vi "oax_gsOrder Analyzer.vi"() -> ()   [LabVIEW 2017]
doc: "This VI provides Gabor order track, which can extract order from sound / vibration signal and playback on multimedia devices. This VI also provides access to Order Map.vi, which displays spectral maps, in menu bar window>> Show Order Map."
uses:
  <vilib>/addons/Sound and Vibration/Order Analysis/Ref Gabor Order Tracking/window information.ctl
  <vilib>/Analysis/1siggen.llb/Ramp Pattern by Samples.vi
  <vilib>/Waveform/WDTFileIO.llb/ Write Waveforms to File (1D).vi
  <vilib>/Waveform/WDTFileIO.llb/Export Waveforms To Spreadsheet File (1D).vi
  <vilib>/addons/Sound and Vibration/Order Analysis/Example Support/Demo VI/Start-Up Kit/OAT Start/global variable.vi
  <vilib>/addons/Sound and Vibration/Order Analysis/Ref Gabor Order Tracking/Get Freq-Time Spectral Map (U8).vi
  <vilib>/addons/Sound and Vibration/Order Analysis/Gabor Order Tracking/SoundVib_Gabor.lvlib
  <vilib>/Analysis/NI_AALBase.lvlib
panel:
  in  "Select Data":string(tree)="Runup.bin"
  in  "Campbell Diagram":bool
  in  "order map":bool
  in  "Save Orders":bool
  in  "Clear":bool
  in  "Delete":bool
  out "Speed at\nCursor (RPM)":dbl
  out "Time at\nCursor (sec)":dbl format="%.2f"
  in  "last path":path
  in  "unit":u16(ring) items=["Order", "Hz"]
  out "window information":T1={"window type"=3, "window length"=1} {"window type" items=["None"=0, "Hanning"=1, "Hamming"=2, "Blackman-Harris"=3, "Exact Blackman"=4, "Blackman"=5, "Flat Top"=6, "4 Term B-Harris"=7, "7 Term B-Harris"=8, "Low Sidelobe"=9, "Gaussian"=62]; "window length" min=0}
  out "TF Plot":u8[][](graph) caption="Time-Frequency Plot"
  out "Cursor Position":cluster{"Cursor X":dbl, "Cursor Y":dbl}={"Cursor X"=347.3140311804009, "Cursor Y"=0.0} {"Cursor Y" format="%.2f"; "Cursor X" format="%.2f"}
  in  "Play Sound":T2(ring)
  in  "Order List":i32[](listbox)
  out "Spectrum":cluster{dbl[], "X":dbl[]}(graph)
  out "mask":bool[][](array[boolean])
  in  "Bandwidth":dbl(slide)=0.5 min=0.0 scale=0.0..1.0 scale format="%.2f"
  in  "extract":bool
  out "X":dbl[](array[numeric]) format="%.2f"
  in  "Selected Order":dbl min=0.0 step=0.10000000149011612 format="%.1f"
  out "Window \nLength":i32
  out "Status":string="Waiting..."
  out "Sample \nRate (Hz)":dbl
  out "File Name":string
  out "S&V plot":dbl[][](graph)
  # "Show Other Formats"
  # "Extract Order Waveforms"
  # "Narrow"
  # "Wide"
  # "Status"
  # "Data Info"
  # "Cursor Values"
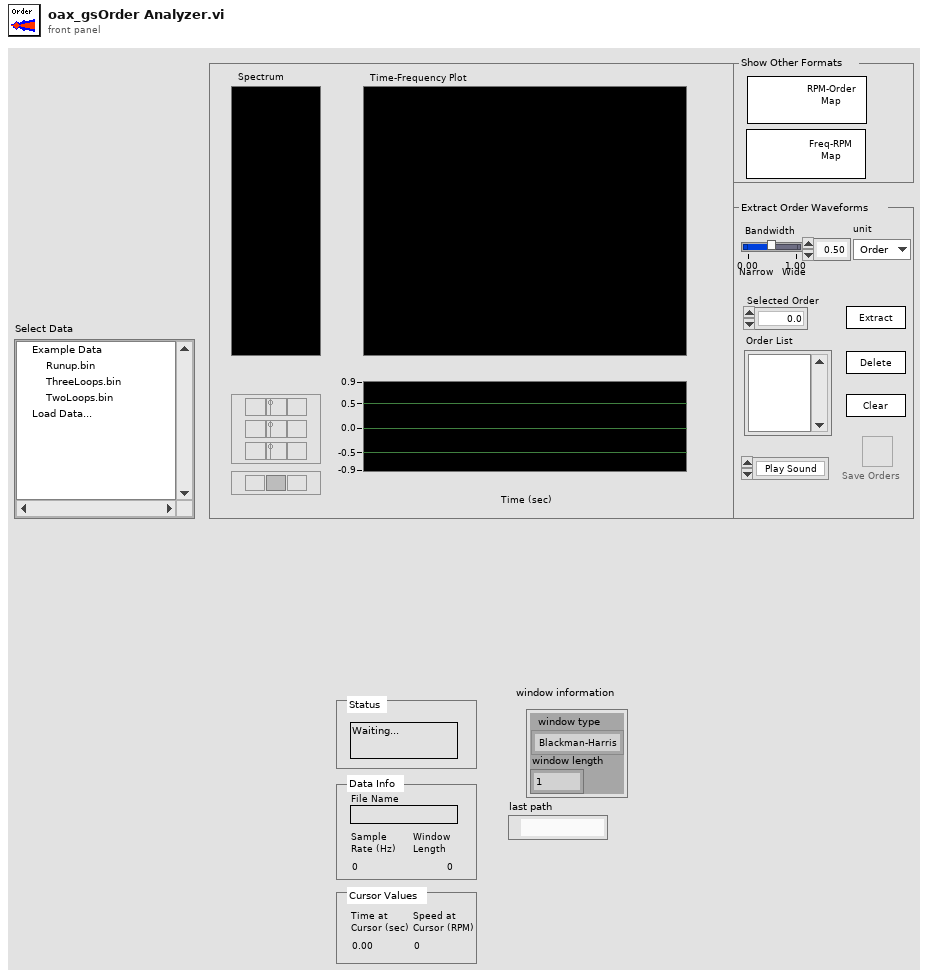
[diagram p1: front panel]
types:
  T1 = typedef "SoundVib_Gabor.lvlib/window information.ctl" = cluster{"window type":u32, "window length":i32}
  T2 = enum16{"Play Sound", "Original Signal", "Selected Orders", "Without Orders"}
  T3 = enum16{"Play Sound", "Original Samples", "Selected Orders", "Without Orders"}
  T4 = typedef "LVPointDoubleTypeDef.ctl" = cluster{"Cursor X":dbl, "Cursor Y":dbl}
  T5 = cluster{"Selected Order":dbl, "Bandwidth":dbl, "unit":u16}
  T6 = typedef "LVRangeTypeDef.ctl" = cluster{"Minimum":dbl, "Maximum":dbl, "Increment":dbl, "Minor Increment":dbl, "Start":dbl}
  T7 = typedef "SoundVib_Gabor.lvlib/GT RefNum.ctl" = refnum<k1>
  T8 = typedef "SoundVib_TachProcess.lvlib/speed profile.ctl" = cluster{"time [s]":dbl[], "speed [RPM]":dbl[]}
  T9 = cluster{"quality":enum16{"mono", "stereo"}, u32, "bits/sample":enum16{"8 bit", "16 bit"}}
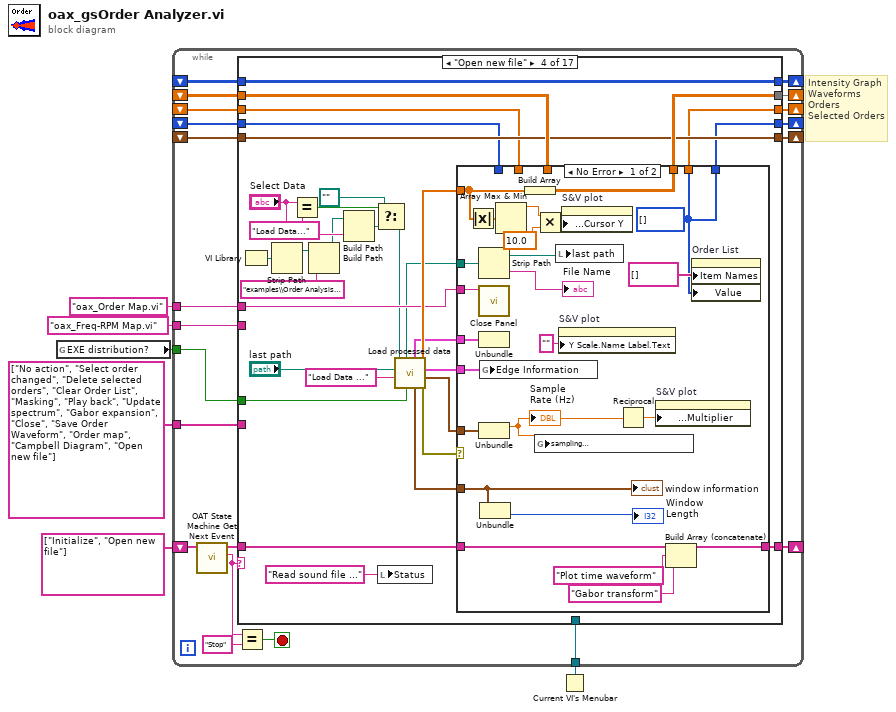
[diagram p0: block diagram]
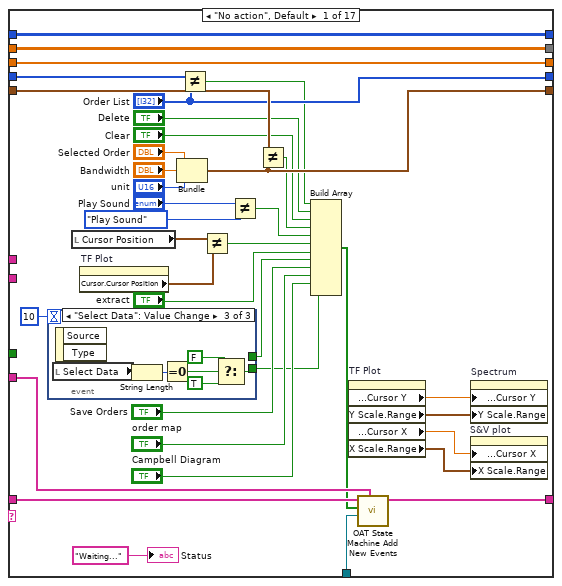
[diagram p2: hidden frame]
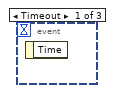
[diagram p3: hidden frame]
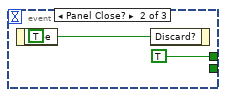
[diagram p4: hidden frame]
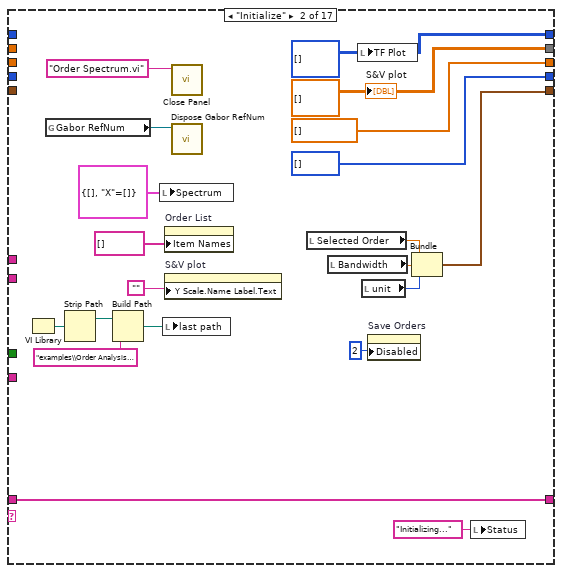
[diagram p5: hidden frame]
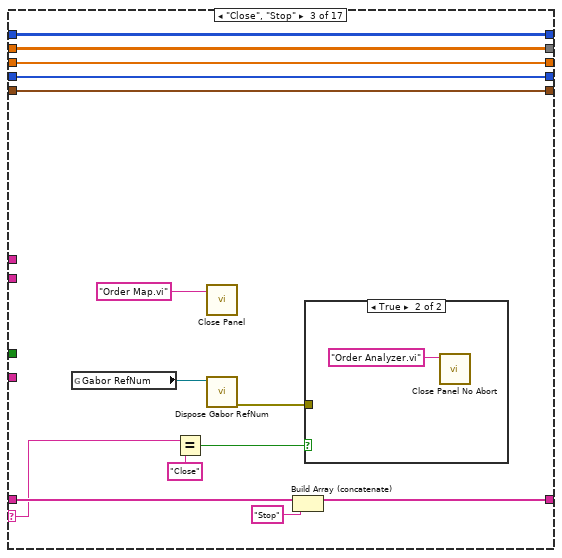
[diagram p6: hidden frame]
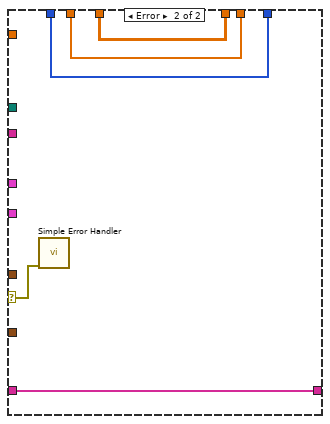
[diagram p8: hidden frame]
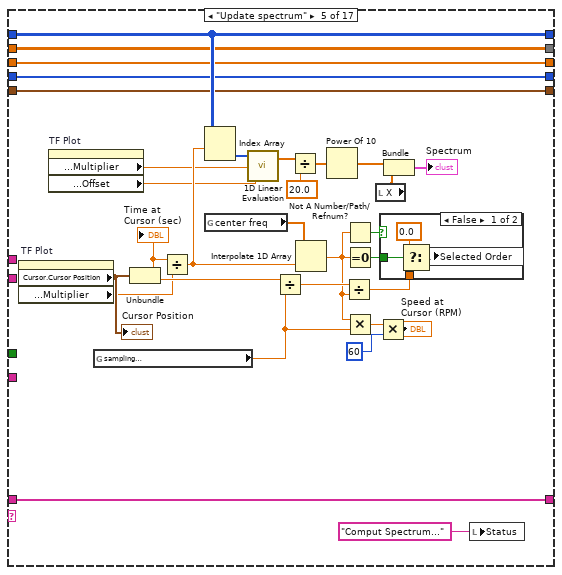
[diagram p9: hidden frame]
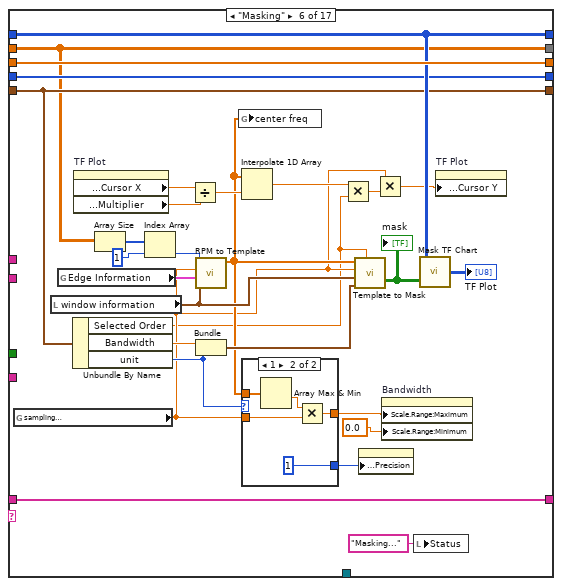
[diagram p11: hidden frame]
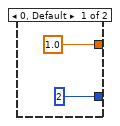
[diagram p12: hidden frame]
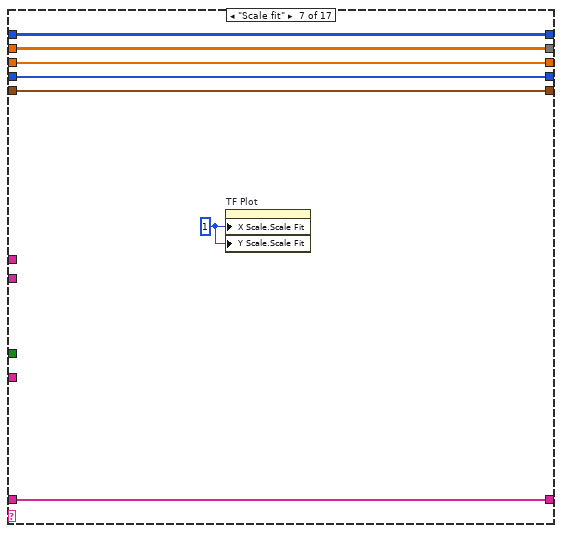
[diagram p13: hidden frame]
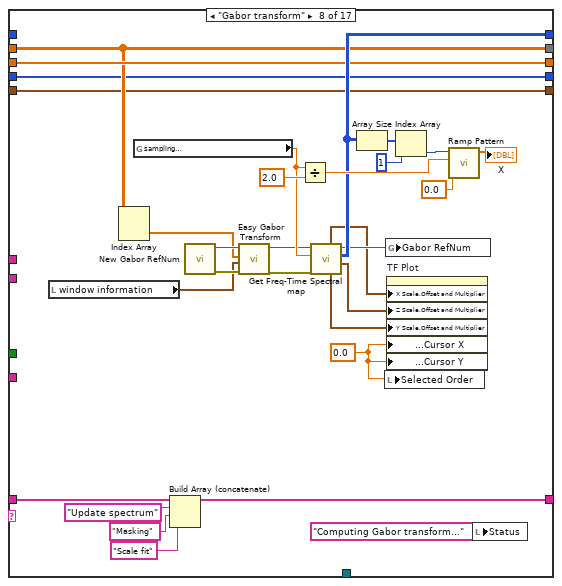
[diagram p14: hidden frame]
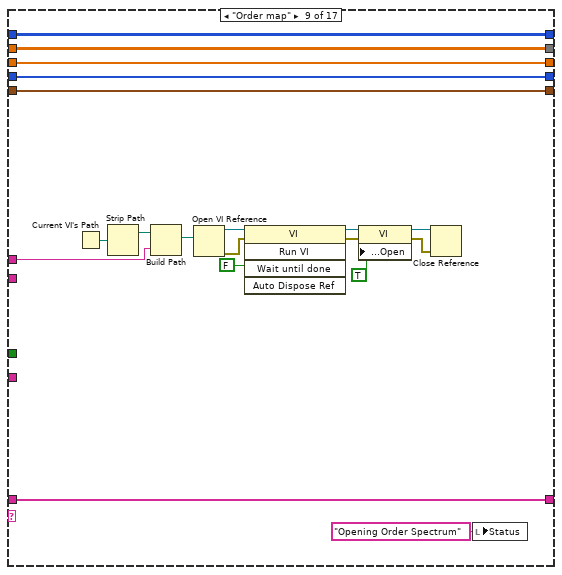
[diagram p15: hidden frame]
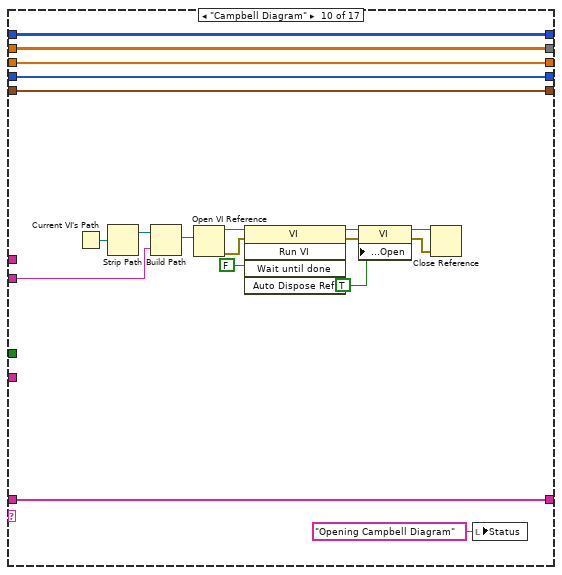
[diagram p16: hidden frame]
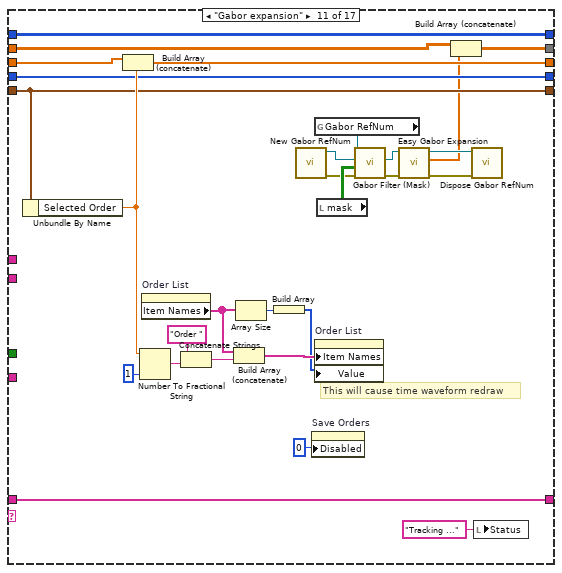
[diagram p17: hidden frame]
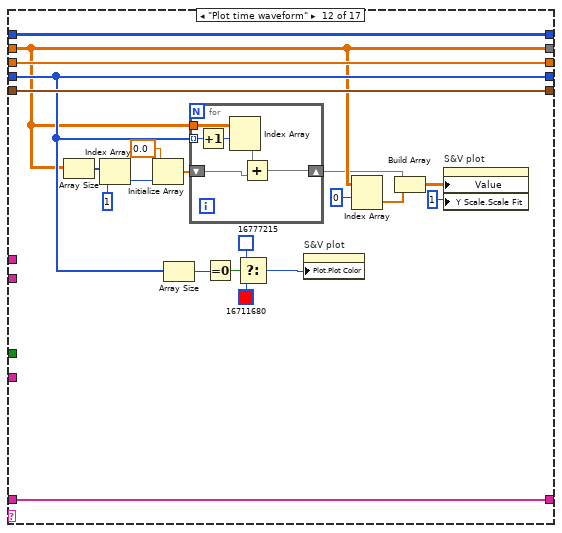
[diagram p18: hidden frame]
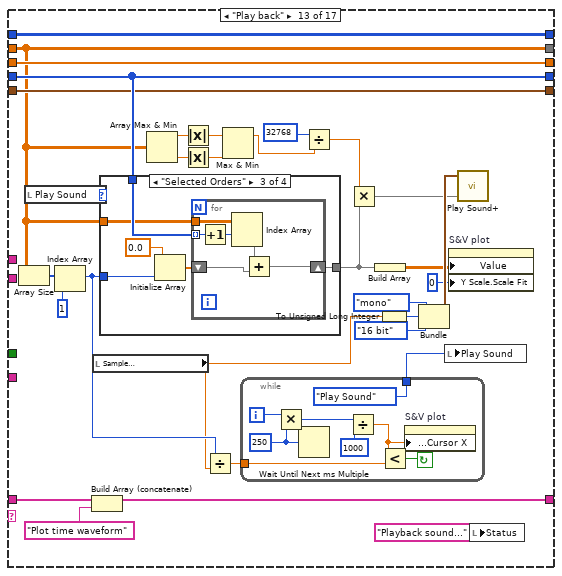
[diagram p19: hidden frame]
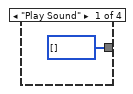
[diagram p20: hidden frame]
diagram:
  # "Intensity Graph\nWaveforms\nOrders\nSelected Orders"
  n1 = global read "global variable.vi" "EXE distribution?"() -> (w2:bool)
  n2 = Current VI's Menubar() -> (w4:refnum<k9>)
  n3 = while {
    tunnel: "oax_Freq-RPM Map.vi" ("VI name") -> [w7]
    tunnel: w2 -> [w8]
    tunnel: "oax_Order Map.vi" ("VI name") -> [w9]
    shift-left: _ -> [w11]
    shift-right: [w10] -> _
    shift-left: _ -> [w12]
    shift-right: [w13] -> _
    tunnel: w4 -> [w14]
    tunnel: string[] ["No action", "Select order changed", "Delete selected orders", "Clear Order List", "Masking", "Play back", "Update spectrum", "Gabor expansion", "Close", "Save Order Waveform", "Order map", "Campbell Diagram", "Open new file"] ("Event Queue Out") -> [w18]
    shift-left: string[] ["Initialize", "Open new file"] ("Event Queue Out") -> [w21]
    shift-right: [w19] -> _
    shift-left: _ -> [w22]
    shift-right: [w24] -> _
    shift-left: _ -> [w23]
    shift-right: [w25] -> _
    shift-left: _ -> [w26]
    shift-right: [w27] -> _
    stop <- w15 stop-if-true
    n4 = call <vilib>:"OAT State Machine Get Next Event.vi"("event queue in"=w21) -> ("next event"=w17:string, "event queue out"=w20:string[])  [unwired: 5 in]
    n5 = Equal?(x=w17, y="Stop" ("item tag")) -> (x = y?=w15:bool)
    n6 = case shown="\"Open new file\"" w17 {
      selector: w17 -> [_ _ w98 _ _ _ _ _ _ _ _ _ _ _ _ _ _]
      tunnel: [w64 w89 w106 w139 w199 w230 w243 w268 w295 w314 w339 w363 w400 w449 w466 w486 w498] -> w27
      tunnel: w26 -> [w64 _ w106 w139 w199 w230 w243 _ w295 w314 w339 w363 w400 w449 w466 w486 w498]
      tunnel: [w63 w80 w105 w135 w198 w223 w242 w265 w294 w313 w337 w347 w377 w443 w457 w485 w492] -> w25
      tunnel: [w62 dbl[] [] w104 w121 w197 w232 w246 w267 w293 w312 w329 w350 w399 w438 w455 w484 w497] -> w24
      tunnel: w23 -> [w63 _ w105 w134 w198 w223 w242 w265 w294 w313 w338 w347 w377 w444 w460 w485 w492]
      tunnel: w22 -> [w62 _ w104 w123 w197 w232 w246 w267 w293 w312 w335 w350 w399 _ w456 w484 w497]
      tunnel: w20 -> [w61 w86 w101 w131 w196 w211 w240 w262 w291 w310 w316 w357 w393 w448 w463 w480 w495]
      tunnel: [w60 w86 w94 w132 w196 w211 w240 w261 w291 w310 w316 w357 w391 w445 w462 w479 w495] -> w19
      tunnel: w18 -> [w59 _ _ _ _ _ _ _ _ _ _ _ _ _ _ _ _]
      tunnel: w14 -> [w57 _ _ _ _ _ _ _ _ _ _ _ _ _ _ _ _]
      tunnel: [w56 w81 w102 w130 w193 w226 w245 w256 w288 w307 w321 w356 w381 w442 w465 w482 w496] -> w13
      tunnel: w12 -> [w55 _ w102 w130 w193 w226 w245 w256 w288 w307 w321 w356 w381 w442 w465 w482 w496]
      tunnel: w11 -> [w36 _ w103 w122 w194 w225 w244 w257 w289 w308 w322 w348 w389 w441 w459 w483 w491]
      tunnel: ["Order List" i32[] [] ("Order List") w103 w120 w194 w225 w244 w257 w289 w308 w322 w348 w389 w441 i32[] [] ("Order List") w483 w491] -> w10
      tunnel: w9 -> [_ _ _ w125 _ _ _ _ w277 _ _ _ _ _ _ _ _]
      tunnel: w8 -> [_ _ _ w119 _ _ _ _ _ _ _ _ _ _ _ _ _]
      tunnel: w7 -> [_ _ _ _ _ _ _ _ _ w296 _ _ _ _ _ _ _]
      frame "No action", Default {
        n7 = event shown="[2] \"Select Data\": Value Change" {
          selector: _ -> [_ _ _]
          dyn-events: _ -> [_ _ _]
          timeout: 10 -> [_ _ _]
          tunnel: [_ TRUE _] -> w32
          tunnel: [_ _ w68] -> w28
          event Timeout {
            n8 = event-data() -> ()  [unwired: 1 in, 1 out]
          }
          event Panel Close? {
            n9 = event-data() -> ()  [unwired: 1 in, 1 out]
            n10 = event-data("Discard?"=TRUE) -> ()  [unwired: 1 in, 1 out]
          }
          event "Select Data": Value Change {
            n11 = local read "Select Data"() -> (w72:string)
            n12 = event-data() -> ()  [unwired: 1 in, 2 out]
            n13 = String Length(string=w72) -> (length=w71:i32)
            n14 = Equal To 0?(x=w71) -> (x = 0?=w70:bool)
            n15 = Select(t=FALSE, s=w70, f=TRUE) -> (s? t:f=w68:bool)
          }
        }
        n16 = local read "Cursor Position"() -> (w53:cluster{"Cursor X":dbl, "Cursor Y":dbl})
        n17 = property on="TF Plot" class="IntGraph (strict)"() -> ("Cursor.Cursor Position"=w52:T4)  [unwired: 2 in, 2 out]
        n18 = Bundle("Selected Order"="Selected Order", "Bandwidth"="Bandwidth", "unit"="unit") -> (w56:T5)  [unwired: 1 in]
        n19 = Not Equal?(x=w36, y="Order List") -> (x != y?=w34:bool)
        n20 = Not Equal?(x=w53, y=w52) -> (x != y?=w45:bool)
        n21 = Not Equal?(x="Play Sound", y=T3."Play Sound" ("play sound")) -> (x != y?=w42:bool)
        n22 = Not Equal?(x=w55, y=w56) -> (x != y?=w46:bool)
        n23 = Build Array(w34, "Delete", "Clear", w46, w42, w45, "extract", w32, "Save Orders", "order map", "Campbell Diagram", w28) -> (w54:bool[])
        n24 = property on="TF Plot" class="IntGraph (strict)"() -> ("Cursor.Cursor Position:Cursor Y"=w49:dbl, "Y Scale.Range"=w50:T6, "Cursor.Cursor Position:Cursor X"=w39:dbl, "X Scale.Range"=w40:T6)  [unwired: 2 in, 2 out]
        n25 = call <vilib>:"OAT State Machine Add New Events.vi"("Event Names"=w59, "Menu Refnum"=w57, "New Events"=w54, "Event Queue In"=w61) -> ("Event Queue Out"=w60:string[])  [unwired: 7 in]
        n26 = property on="Spectrum" class="XYGraph (strict)"("Cursor.Cursor Position:Cursor Y"=w49, "Y Scale.Range"=w50) -> ()  [unwired: 2 in, 2 out]
        n27 = property on="S&V plot" class="WFGraph (strict)"("Cursor.Cursor Position:Cursor X"=w39, "X Scale.Range"=w40) -> ()  [unwired: 2 in, 2 out]
        "Status" <- "Waiting..." ("status")
      }
      frame "Initialize" {
        w80 = dbl[][] []
        w89 = u8[][] [] ("graph [U8]")
        n28 = VI Library() -> (path=w78:path)
        n29 = global read "global variable.vi" "Gabor RefNum"() -> (w90:T7)
        n30 = Strip Path(path=w78) -> (stripped path=w77:path)  [unwired: 1 out]
        n31 = Build Path(base path=w77, name or relative path="examples\\Order Analysis\\Demo VI\\Example Data") -> (appended path=w75:path)
        n32 = local write "Spectrum"(cluster{dbl[], "X":dbl[]} {[], "X"=[]} ("Instantaneous\nSpectrum")) -> ()
        n33 = local write "last path"(w75) -> ()
        n34 = property on="Order List" class="LstBox (strict)"("Item Names"=string[] [] ("Write Attribute")) -> ()  [unwired: 2 in, 2 out]
        n35 = property on="S&V plot" class="WFGraph (strict)"("Y Scale.Name Label.Text"="") -> ()  [unwired: 2 in, 2 out]
        n36 = call <vilib>:"Close Panel.vi"("VI name"="Order Spectrum.vi") -> ()  [unwired: 10 in, 1 out]
        n37 = call <vilib>:"Dispose Gabor RefNum.vi"("RefNum in"=w90) -> ()  [unwired: 7 in, 1 out]
        n38 = local read "Selected Order"() -> (w83:dbl)
        n39 = local read "Bandwidth"() -> (w82:dbl)
        n40 = local write "TF Plot"(w89) -> ()
        n41 = local read "unit"() -> (w79:u16)
        n42 = property on="Save Orders" class="Bool"("Disabled"=u8 2) -> ()  [unwired: 2 in, 2 out]
        n43 = Bundle("Selected Order"=w83, "Bandwidth"=w82, "unit"=w79) -> (w81:T5)  [unwired: 1 in]
        n44 = local write "Status"("Initializing..." ("status")) -> ()
        "S&V plot" <- w80
      }
      frame "Close", "Stop" {
        n45 = global read "global variable.vi" "Gabor RefNum"() -> (w100:T7)
        n46 = Equal?(x=w98, y="Close") -> (x = y?=w96:bool)
        n47 = call <vilib>:"Close Panel.vi"("VI name"="Order Map.vi") -> ()  [unwired: 10 in, 1 out]
        n48 = call <vilib>:"Dispose Gabor RefNum.vi"("RefNum in"=w100) -> ("error out"=w95:errorcluster)  [unwired: 7 in]
        n49 = Build Array (concatenate)(w101, "Stop") -> (w94:string[])
        n50 = case shown="True" w96 {
          tunnel: w95 -> [_ _]
          frame False {
          }
          frame True {
            n51 = call <vilib>:"Close Panel No Abort.vi"("VI name"="Order Analyzer.vi") -> ()  [unwired: 10 in, 1 out]
          }
        }
      }
      frame "Open new file" {
        n52 = VI Library() -> (path=w111:path)
        n53 = Strip Path(path=w111) -> (stripped path=w110:path)  [unwired: 1 out]
        n54 = Equal?(x="Select Data", y="Load Data...") -> (x = y?=w114:bool)
        n55 = Build Path(base path=w110, name or relative path="examples\\Order Analysis\\Demo VI\\Example Data") -> (appended path=w108:path)
        n56 = Build Path(base path=w108, name or relative path="Select Data") -> (appended path=w113:path)
        n57 = Select(t=path "" ("last path"), s=w114, f=w113) -> (s? t:f=w112:path)
        n58 = local write "Status"("Read sound file ..." ("status")) -> ()
        n59 = call <vilib>:"Load processed data.vi"("EXE distribution?"=w119, "Prompt"="Load Data ...", "start path"="last path", "file path"=w112) -> ("error out"=w136:errorcluster, "parameters"=w127:cluster{"sample rate":sgl, "pulses/rev":i32}, "speed profile"=w138:T8, "S&V samples"=w129:dbl[], "window info"=w126:T1, "lables"=w128:cluster{"tach lable":string, "S&V lable":string}, "file path out"=w124:path)  [unwired: 1 in]
        n60 = case shown="No Error" w136 {
          selector: w136 -> [_ w166]
          tunnel: w124 -> [w161 _]
          tunnel: w138 -> [w160 _]
          tunnel: w127 -> [w155 _]
          tunnel: w129 -> [w145 _]
          tunnel: [w158 w168] -> w135
          tunnel: w134 -> [_ w168]
          tunnel: [w157 w167] -> w132
          tunnel: w131 -> [w156 w167]
          tunnel: w128 -> [w153 _]
          tunnel: w126 -> [w150 _]
          tunnel: w125 -> [w163 _]
          tunnel: w123 -> [_ w165]
          tunnel: w122 -> [_ w164]
          tunnel: [w146 w165] -> w121
          tunnel: [w146 w164] -> w120
          frame No Error {
            w146 = i32[] [] ("Order List")
            n61 = Absolute Value(x=w145) -> (abs(x)=w144:dbl[])
            n62 = Strip Path(path=w161) -> (stripped path=w148:path, name=→"File Name":string)
            n63 = call <vilib>:"Close Panel.vi"("VI name"=w163) -> ()  [unwired: 10 in, 1 out]
            n64 = Unbundle(w153) -> ()  [unwired: 2 out]
            n65 = Unbundle(w155) -> ("sample rate"=w154:sgl)  [unwired: 1 out]
            "Sample \nRate (Hz)" <- w154
            n66 = global write "global variable.vi" "Edge Information"(w160) -> ()
            n67 = Unbundle(w150) -> ("window length"=→"Window \nLength":i32)  [unwired: 1 out]
            n68 = Array Max & Min(array=w144) -> (max value=w143:dbl)  [unwired: 3 out]
            n69 = Build Array(w145) -> (w158:dbl[][])
            n70 = Multiply(x=w143, y=10.0) -> (x*y=w141:dbl)
            n71 = global write "global variable.vi" "sampling \nfrequency (Hz)"(w154) -> ()
            n72 = local write "last path"(w148) -> ()
            n73 = property on="S&V plot" class="WFGraph (strict)"("Y Scale.Name Label.Text"="") -> ()  [unwired: 2 in, 2 out]
            n74 = property on="S&V plot" class="WFGraph (strict)"("Cursor.Cursor Position:Cursor Y"=w141) -> ()  [unwired: 2 in, 2 out]
            n75 = Reciprocal(x=w154) -> (1/x=w159:sgl)
            n76 = property on="S&V plot" class="WFGraph (strict)"("X Scale.Offset and Multiplier:Multiplier"=w159) -> ()  [unwired: 2 in, 2 out]
            n77 = Build Array (concatenate)(w156, "Plot time waveform" ("status"), "Gabor transform" ("status")) -> (w157:string[])
            n78 = property on="Order List" class="LstBox (strict)"("Item Names"=string[] [], "Value"=w146) -> ()  [unwired: 2 in, 2 out]
            "window information" <- w150
          }
          frame Error {
            n79 = call <vilib>:"Simple Error Handler.vi"("error in (no error)"=w166) -> ()  [unwired: 4 in, 5 out]
          }
        }
      }
      frame "Update spectrum" {
        n80 = property on="TF Plot" class="IntGraph (strict)"() -> ("Cursor.Cursor Position"=w187:T4, "X Scale.Offset and Multiplier:Multiplier"=w184:dbl)  [unwired: 2 in, 2 out]
        "Cursor Position" <- w187
        n81 = property on="TF Plot" class="IntGraph (strict)"() -> ("Z Scale.Offset and Multiplier:Multiplier"=w179:dbl, "Z Scale.Offset and Multiplier:Offset"=w178:dbl)  [unwired: 2 in, 2 out]
        n82 = global read "global variable.vi" "sampling \nfrequency (Hz)"() -> (w171:dbl)
        n83 = Unbundle(w187) -> ("Cursor X"=w173:dbl, "Cursor Y"=w186:dbl)
        "Time at\nCursor (sec)" <- w173
        n84 = Divide(x=w173, y=w184) -> (x/y=w185:dbl)
        n85 = Index Array(array=w199, index (row)=w185) -> (element=w183:u8[])  [unwired: 1 in]
        n86 = global read "global variable.vi" "center freq"() -> (w177:dbl[])
        n87 = call <vilib>:"1D Linear Evaluation.vi"("offset"=w178, "scale"=w179, "X"=w183) -> ("Y[i]=X[i]*a+b"=w182:dbl[])  [unwired: 1 out]
        n88 = Divide(x=w186, y=w171) -> (x/y=w189:dbl)
        n89 = Divide(x=w182, y=20.0 ("Write Attribute")) -> (x/y=w181:dbl[])
        n90 = Interpolate 1D Array(1:w185, 2:w177) -> (0:w176:dbl)
        n91 = Power Of 10(x=w181) -> (10^x=w190:dbl[])
        n92 = Divide(x=w189, y=w176) -> (x/y=w188:dbl)
        n93 = Not A Number/Path/Refnum?(number/path/refnum=w176) -> (NaN/Path/Refnum?=w169:bool)
        n94 = Equal To 0?(x=w176) -> (x = 0?=w170:bool)
        n95 = Multiply(x=w176, y=w171) -> (x*y=w172:dbl)
        n96 = local read "X"() -> (w191:dbl[])
        n97 = Multiply(x=w172, y=60) -> (x*y=→"Speed at\nCursor (RPM)":dbl)
        n98 = case shown="False" w169 {
          tunnel: w188 -> [w203 _]
          tunnel: w170 -> [w200 _]
          frame False {
            n99 = Select(t=0.0, s=w200, f=w203) -> (s? t:f=w201:dbl)
            n100 = local write "Selected Order"(w201) -> ()
          }
          frame True {
          }
        }
        n101 = Bundle(w190, "X"=w191) -> (→"Spectrum":cluster{dbl[], "X":dbl[]})  [unwired: 1 in]
        n102 = local write "Status"("Comput Spectrum..." ("status")) -> ()
      }
      frame "Masking" {
        n103 = global read "global variable.vi" "sampling \nfrequency (Hz)"() -> (w209:dbl)
        n104 = local read "window information"() -> (w218:T1)
        n105 = global read "global variable.vi" "Edge Information"() -> (w224:T8)
        n106 = Unbundle By Name(w226) -> ("Selected Order"=w208:dbl, "Bandwidth"=w217:dbl, "unit"=w216:u16)
        n107 = property on="TF Plot" class="IntGraph (strict)"() -> ("Cursor.Cursor Position:Cursor X"=w231:dbl, "X Scale.Offset and Multiplier:Multiplier"=w227:dbl)  [unwired: 2 in, 2 out]
        n108 = Array Size(array=w223) -> (size(s)=w222:i32[])
        n109 = Index Array(array=w222, index=1 ("Index")) -> (element=w221:i32)
        n110 = Divide(x=w231, y=w227) -> (x/y=w228:dbl)
        n111 = call <vilib>:"RPM to Template.vi"("window info"=w218, "speed profile"=w224, "sampling frequency [Hz]"=w209, "signal length"=w221) -> ("Gabor template"=w214:dbl[])  [unwired: 6 in, 1 out]
        n112 = Bundle("Bandwidth"=w217, "unit"=w216) -> (w215:cluster{"Bandwidth":dbl, "unit":u16})  [unwired: 1 in]
        n113 = global write "global variable.vi" "center freq"(w214) -> ()
        n114 = Interpolate 1D Array(1:w228, 2:w214) -> (0:w220:dbl)
        n115 = case shown="1" w216 {
          tunnel: w214 -> [_ w239]
          tunnel: w209 -> [_ w237]
          tunnel: [1.0 w236] -> w213
          tunnel: [u8 2 u8 1] -> w212
          frame 0, Default {
          }
          frame 1 {
            n116 = Array Max & Min(array=w239) -> (min value=w238:dbl)  [unwired: 3 out]
            n117 = Multiply(x=w238, y=w237) -> (x*y=w236:dbl)
          }
        }
        n118 = Multiply(x=w220, y=w208) -> (x*y=w204:dbl)
        n119 = call <vilib>:"Template to Mask.vi"("order (1.0)"=w208, "bandwidth"=w215, "window info"=w218, "sampling frequency [S/s]"=w209, "Gabor template"=w214) -> ("mask array"=w206:bool[][])  [unwired: 6 in]
        "mask" <- w206
        n120 = property class="DigNum (strict)"("Format & Precision:Precision"=w212) -> ()  [unwired: 2 in, 2 out]
        n121 = Multiply(x=w209, y=w204) -> (x*y=w207:dbl)
        n122 = property on="Bandwidth" class="Slide (strict)"("Scale.Range:Maximum"=w213, "Scale.Range:Minimum"=0.0) -> ()  [unwired: 2 in, 2 out]
        n123 = local write "Status"("Masking..." ("status")) -> ()
        n124 = call <vilib>:"Mask TF Chart.vi"("Mask Array"=w206, "TF plot"=w230) -> ("TF plot Out"=→"TF Plot":u8[][])
        n125 = property on="TF Plot" class="IntGraph (strict)"("Cursor.Cursor Position:Cursor Y"=w207) -> ()  [unwired: 2 in, 2 out]
      }
      frame "Scale fit" {
        w241 = u8 1 ("X Scale.Scale Fit")
        n126 = property on="TF Plot" class="IntGraph (strict)"("X Scale.Scale Fit"=w241, "Y Scale.Scale Fit"=w241) -> ()  [unwired: 2 in, 2 out]
      }
      frame "Gabor transform" {
        w247 = 0.0
        n127 = local read "window information"() -> (w255:T1)
        n128 = Index Array(array=w265) -> (element=w263:dbl[])  [unwired: 2 in]
        n129 = global read "global variable.vi" "sampling \nfrequency (Hz)"() -> (w254:dbl)
        n130 = Build Array (concatenate)(w262, "Update spectrum" ("status"), "Masking" ("status"), "Scale fit" ("status")) -> (w261:string[])
        n131 = call <vilib>:"New Gabor RefNum.vi"() -> ("error out"=w264:errorcluster, "RefNum"=w276:T7)  [unwired: 9 in]
        n132 = call <vilib>:"Easy Gabor Transform.vi"("error in (no error)"=w264, "window info"=w255, "x[n]"=w263, "RefNum in"=w276) -> ("error out"=w275:errorcluster, "RefNum out"=w253:T7)  [unwired: 3 in, 3 out]
        n133 = Divide(x=w254, y=2.0) -> (x/y=w270:dbl)
        n134 = call-poly <vilib>:"Get Freq-Time Spectral map.vi"("error in (no error)"=w275, "sampling frequency [Hz]"=w254, "RefNum in"=w253) -> ("quantization info"=w250:cluster{"offset":dbl, "multiplier":dbl}, "spectral map"=w268:u8[][], "RefNum out"=w266:T7, "frequency scale"=w249:cluster{"offset":dbl, "multiplier":dbl}, "time scale"=w251:cluster{"offset":dbl, "multiplier":dbl})  [unwired: 3 in, 1 out]
        n135 = Array Size(array=w268) -> (size(s)=w274:i32[])
        n136 = local write "Selected Order"(w247) -> ()
        n137 = global write "global variable.vi" "Gabor RefNum"(w266) -> ()
        n138 = property on="TF Plot" class="IntGraph (strict)"("X Scale.Offset and Multiplier"=w251, "Z Scale.Offset and Multiplier"=w250, "Y Scale.Offset and Multiplier"=w249, "Cursor.Cursor Position:Cursor X"=w247, "Cursor.Cursor Position:Cursor Y"=w247) -> ()  [unwired: 2 in, 2 out]
        n139 = Index Array(array=w274, index=1 ("Index")) -> (element=w272:i32)
        n140 = call-poly <vilib>:"Ramp Pattern.vi"("start"=0.0, "end"=w270, "samples"=w272) -> ("Ramp Pattern"=→"X":dbl[])  [unwired: 7 in, 1 out]
        n141 = local write "Status"("Computing Gabor transform..." ("status")) -> ()
      }
      frame "Order map" {
        n142 = Current VI's Path() -> (path=w292:path)
        n143 = Strip Path(path=w292) -> (stripped path=w287:path)  [unwired: 1 out]
        n144 = Build Path(base path=w287, name or relative path=w277) -> (appended path=w286:path)
        n145 = Open VI Reference(vi path=w286) -> (vi reference=w285:refnum<vi>, error out=w284:errorcluster)  [unwired: 5 in]
        n146 = invoke class="VI" method="Run VI"(reference=w285, error in=w284, "Wait until done"=FALSE) -> (reference out=w282:refnum<vi>, error out=w281:errorcluster)  [unwired: 2 in, 3 out]
        n147 = property class="VI"(reference=w282, error in=w281, "Front Panel Window:Open"=TRUE) -> (reference out=w278:refnum<vi>, error out=w279:errorcluster)
        n148 = Close Reference(reference=w278, error in (no error)=w279) -> ()  [unwired: 1 out]
        n149 = local write "Status"("Opening Order Spectrum" ("status")) -> ()
      }
      frame "Campbell Diagram" {
        n150 = Current VI's Path() -> (path=w311:path)
        n151 = Strip Path(path=w311) -> (stripped path=w306:path)  [unwired: 1 out]
        n152 = Build Path(base path=w306, name or relative path=w296) -> (appended path=w305:path)
        n153 = Open VI Reference(vi path=w305) -> (vi reference=w304:refnum<vi>, error out=w303:errorcluster)  [unwired: 5 in]
        n154 = invoke class="VI" method="Run VI"(reference=w304, error in=w303, "Wait until done"=FALSE) -> (reference out=w301:refnum<vi>, error out=w300:errorcluster)  [unwired: 2 in, 3 out]
        n155 = property class="VI"(reference=w301, error in=w300, "Front Panel Window:Open"=TRUE) -> (reference out=w297:refnum<vi>, error out=w298:errorcluster)
        n156 = Close Reference(reference=w297, error in (no error)=w298) -> ()  [unwired: 1 out]
        n157 = local write "Status"("Opening Campbell Diagram" ("status")) -> ()
      }
      frame "Gabor expansion" {
        # "This will cause time waveform redraw"
        n158 = Unbundle By Name(w321) -> ("Selected Order"=w323:dbl)
        n159 = Build Array (concatenate)(w335, w323) -> (w329:dbl[])
        n160 = Number To Fractional String(number=w323, precision (6)=i16 1) -> (F-format string=w333:string)  [unwired: 2 in]
        n161 = property on="Order List" class="LstBox (strict)"() -> ("Item Names"=w319:string[])  [unwired: 2 in, 2 out]
        n162 = Concatenate Strings("Order " ("Substring"), w333) -> (w330:string)
        n163 = Build Array (concatenate)(w319, w330) -> (w328:string[])
        n164 = Array Size(array=w319) -> (size(s)=w317:i32)
        n165 = Build Array(w317) -> (w318:i32[])
        n166 = call <vilib>:"New Gabor RefNum.vi"() -> ("error out"=w325:errorcluster, "RefNum"=w341:T7)  [unwired: 9 in]
        n167 = property on="Save Orders" class="Bool"("Disabled"=u8 0) -> ()  [unwired: 2 in, 2 out]
        n168 = global read "global variable.vi" "Gabor RefNum"() -> (w331:T7)
        n169 = property on="Order List" class="LstBox (strict)"("Item Names"=w328, "Value"=w318) -> ()  [unwired: 2 in, 2 out]
        n170 = local read "mask"() -> (w336:bool[][])
        n171 = call <vilib>:"Gabor Filter (Mask).vi"("error in (no error)"=w325, "mask array"=w336, "dest RefNum in"=w341, "src RefNum in"=w331) -> ("error out"=w326:errorcluster, "dest RefNum out"=w342:T7)  [unwired: 5 in, 1 out]
        n172 = call <vilib>:"Easy Gabor Expansion.vi"("error in (no error)"=w326, "RefNum in"=w342) -> ("error out"=w327:errorcluster, "time waveform"=w320:dbl[], "RefNum out"=w340:T7)  [unwired: 7 in]
        n173 = Build Array (concatenate)(w338, w320) -> (w337:dbl[][])
        n174 = call <vilib>:"Dispose Gabor RefNum.vi"("error in (no error)"=w327, "RefNum in"=w340) -> ()  [unwired: 6 in, 1 out]
        n175 = local write "Status"("Tracking ..." ("status")) -> ()
      }
      frame "Plot time waveform" {
        n176 = Array Size(array=w347) -> (size(s)=w353:i32[])
        n177 = Index Array(array=w353, index=1 ("Index")) -> (element=w349:i32)
        n178 = Initialize Array(0.0 ("y"), w349) -> (w346:dbl[])
        n179 = Array Size(array=w348) -> (size(s)=w358:i32)
        n180 = for {
          tunnel: w347 -> [w368]
          tunnel: w348 -> [w367] mode=indexing
          shift-right: [w366] -> w344
          shift-left: w346 -> [w365]
          n181 = Increment(x=w367) -> (x+1=w369:i32)
          n182 = Index Array(array=w368, index (row)=w369) -> (element=w364:dbl[])  [unwired: 1 in]
          n183 = Add(x=w364, y=w365) -> (x+y=w366:dbl[])
        }
        n184 = Equal To 0?(x=w358) -> (x = 0?=w359:bool)
        n185 = Select(t=u32 16777215 ("Read Attribute"), s=w359, f=u32 16711680 ("Read Attribute")) -> (s? t:f=w362:u32)
        n186 = property on="S&V plot" class="WFGraph (strict)"("Plot.Plot Color"=w362) -> ()  [unwired: 2 in, 2 out]
        n187 = Index Array(array=w347, index (row)=0) -> (element=w343:dbl[])  [unwired: 1 in]
        n188 = Build Array(w344, w343) -> (w355:dbl[][])
        n189 = property on="S&V plot" class="WFGraph (strict)"("Value"=w355, "Y Scale.Scale Fit"=u8 1) -> ()  [unwired: 2 in, 2 out]
      }
      frame "Play back" {
        n190 = Array Size(array=w377) -> (size(s)=w376:i32[])
        n191 = local read "Play Sound"() -> (w388:T2)
        n192 = Index Array(array=w376, index=1 ("Index")) -> (element=w375:i32)
        n193 = Build Array (concatenate)(w393, "Plot time waveform" ("status")) -> (w391:string[])
        n194 = local read "Sample \nRate (Hz)"() -> (w374:dbl)
        n195 = case shown="\"Selected Orders\"" w388 {
          tunnel: w389 -> [_ _ w418 w429]
          tunnel: [i16[] [] w410 w417 w428] -> w380
          tunnel: w377 -> [_ w412 w416 w427]
          tunnel: w375 -> [_ _ w413 _]
          frame "Play Sound" {
          }
          frame "Original Signal" {
            n196 = Index Array(array=w412, index (row)=0 ("Index")) -> (element=w410:dbl[])  [unwired: 1 in]
          }
          frame "Selected Orders" {
            n197 = Initialize Array(0.0 ("y"), w413) -> (w415:dbl[])
            n198 = for {
              tunnel: w416 -> [w423]
              tunnel: w418 -> [w422] mode=indexing
              shift-right: [w421] -> w417
              shift-left: w415 -> [w420]
              n199 = Increment(x=w422) -> (x+1=w424:i32)
              n200 = Index Array(array=w423, index (row)=w424) -> (element=w419:dbl[])  [unwired: 1 in]
              n201 = Add(x=w419, y=w420) -> (x+y=w421:dbl[])
            }
          }
          frame "Without Orders" {
            n202 = Index Array(array=w427, index (row)=0 ("Index")) -> (element=w425:dbl[])  [unwired: 1 in]
            n203 = for {
              tunnel: w427 -> [w434]
              tunnel: w429 -> [w433] mode=indexing
              shift-right: [w431] -> w428
              shift-left: w425 -> [w432]
              n204 = Increment(x=w433) -> (x+1=w435:i32)
              n205 = Index Array(array=w434, index (row)=w435) -> (element=w430:dbl[])  [unwired: 1 in]
              n206 = Subtract(x=w432, y=w430) -> (x-y=w431:dbl[])
            }
          }
        }
        n207 = Array Max & Min(array=w377) -> (max value=w387:dbl, min value=w386:dbl)  [unwired: 2 out]
        n208 = Absolute Value(x=w387) -> (abs(x)=w385:dbl)
        n209 = Absolute Value(x=w386) -> (abs(x)=w384:dbl)
        n210 = Divide(x=w375, y=w374) -> (x/y=w398:dbl)
        n211 = Max & Min(x=w385, y=w384) -> (max(x,y)=w382:dbl)  [unwired: 1 out]
        n212 = while {
          tunnel: [T2."Play Sound" ("play sound")] -> w373
          tunnel: w398 -> [w403]
          i -> [w407]
          stop <- w402 continue-if-true
          w406 = u32 250 ("milliseconds to wait")
          n213 = Multiply(x=w407, y=w406) -> (x*y=w408:u32)
          n214 = Wait Until Next ms Multiple(millisecond multiple=w406) -> ()  [unwired: 1 out]
          n215 = Divide(x=w408, y=u32 1000) -> (x/y=w404:dbl)
          n216 = Less?(x=w404, y=w403) -> (x < y?=w402:bool)
          n217 = property on="S&V plot" class="WFGraph (strict)"("Cursor.Cursor Position:Cursor X"=w404) -> ()  [unwired: 2 in, 2 out]
        }
        n218 = Divide(x=32768, y=w382) -> (x/y=w379:dbl)
        n219 = Multiply(x=w379, y=w380) -> (x*y=w378:dbl[])
        n220 = Build Array(w380) -> (w372:dbl[][])
        n221 = To Unsigned Long Integer(number=w374) -> (unsigned 32bit integer=w394:u32)
        n222 = Bundle("quality"=enum16{"mono", "stereo"}."mono", w394, "bits/sample"=enum16{"8 bit", "16 bit"}."16 bit") -> (w397:T9)  [unwired: 1 in]
        n223 = local write "Play Sound"(w373) -> ()
        n224 = property on="S&V plot" class="WFGraph (strict)"("Value"=w372, "Y Scale.Scale Fit"=u8 0) -> ()  [unwired: 2 in, 2 out]
        n225 = call <vilib>:"Play Sound+.vi"("Array"=w378, "sound format"=w397) -> ()  [unwired: 1 in]
        n226 = local write "Status"("Playback sound..." ("status")) -> ()
      }
      frame "Clear Order List" {
        n227 = Build Array (concatenate)(w448, "Plot time waveform" ("status")) -> (w445:string[])
        n228 = Array Subset(array=w444, length (row)=1 ("Index")) -> (w443:dbl[][])  [unwired: 3 in]
        n229 = property on="Order List" class="LstBox (strict)"("Item Names"=string[] [] ("Write Attribute")) -> ()  [unwired: 2 in, 2 out]
        n230 = property on="Save Orders" class="Bool"("Disabled"=u8 2) -> ()  [unwired: 2 in, 2 out]
        n231 = local read "Selected Order"() -> (w437:dbl)
        n232 = Build Array (concatenate)(dbl[] [], w437) -> (w438:dbl[])
      }
      frame "Delete selected orders" {
        n233 = Array Size(array=w459) -> (size(s)=w458:i32)
        n234 = for {
          N: w458 -> [_]
          tunnel: w459 -> [w476]
          shift-right: [w477] -> w457
          shift-left: w460 -> [w478]
          shift-right: [w474] -> _
          shift-left: w458 -> [w475]
          shift-right: [w471] -> w455
          shift-left: w456 -> [w472]
          n235 = property on="Order List" class="LstBox (strict)"() -> ("Item Names"=w469:string[])  [unwired: 2 in, 2 out]
          n236 = Decrement(x=w475) -> (x-1=w474:i32)
          n237 = Index Array(array=w476, index=w474) -> (element=w467:i32)
          n238 = Increment(x=w467) -> (x+1=w473:i32)
          n239 = Delete From Array(array=w469, index=w467) -> (array with subset deleted=w468:string[])  [unwired: 1 in, 1 out]
          n240 = Delete From Array(array=w478, index (row)=w473) -> (array with subset deleted=w477:dbl[][])  [unwired: 2 in, 1 out]
          n241 = Delete From Array(array=w472, length=1, index=w467) -> (array with subset deleted=w471:dbl[])  [unwired: 1 out]
          n242 = property on="Order List" class="LstBox (strict)"("Item Names"=w468) -> ()  [unwired: 2 in, 2 out]
        }
        n243 = Build Array (concatenate)(w463, "Plot time waveform" ("status")) -> (w462:string[])
        n244 = Array Size(array=w455) -> (size(s)=w454:i32)
        n245 = Equal To 0?(x=w454) -> (x = 0?=w453:bool)
        n246 = Select(t=u8 2 ("Disabled"), s=w453, f=u8 0 ("Disabled")) -> (s? t:f=w452:u8)
        n247 = property on="Save Orders" class="Bool"("Disabled"=w452) -> ()  [unwired: 2 in, 2 out]
      }
      frame "Select order changed" {
        n248 = Build Array (concatenate)(w480, "Plot time waveform" ("status")) -> (w479:string[])
      }
      frame "Save Order Waveform" {
        n249 = global read "global variable.vi" "sampling \nfrequency (Hz)"() -> (w494:dbl)
        n250 = Reciprocal(x=w494) -> (1/x=w488:dbl)
        n251 = for {
          tunnel: w492 -> [w510]
          tunnel: w488 -> [w513]
          tunnel: [w511] -> w493 mode=indexing
          tunnel: w491 -> [w509] mode=indexing
          n252 = Increment(x=w509) -> (x+1=w507:i32)
          n253 = Index Array(array=w510, index (row)=w507) -> (element=w508:dbl[])  [unwired: 1 in]
          n254 = Bundle By Name("t0"=timestamp(0 s since 1904-01-01), "dt"=w513, "Y"=w508) -> (w511:waveform(dbl))  [unwired: 1 in]
        }
        n255 = call <vilib>:"Save File Configuration for Order Waveform.vi"() -> ("Cancel 2"=w487:bool, "Path"=w489:path, "binary?"=w490:bool)  [unwired: 9 in]
        n256 = case shown="False" w487 {
          tunnel: w493 -> [w501 _]
          tunnel: w490 -> [w500 _]
          tunnel: w489 -> [w499 _]
          frame False {
            n257 = case shown="False" w500 {
              tunnel: w501 -> [w502 w506]
              tunnel: w499 -> [w503 w504]
              frame False {
                n258 = call-poly <vilib>:"Export Waveforms to Spreadsheet File.vi"("waveforms"=w502, "file path (dialog if empty)"=w503) -> ()  [unwired: 8 in, 2 out]
              }
              frame True {
                n259 = call-poly <vilib>:"Write Waveforms to File.vi"("append to file? (new file:F)"=FALSE, "waveform array"=w506, "file path (dialog if empty)"=w504) -> ()  [unwired: 7 in, 2 out]
              }
            }
          }
          frame True {
          }
        }
      }
    }
  }
